vi "LIA Select Decimator.vi"(5 "lock-in.decimator1 0":enum16{"None", "FIR"}(ring), 7 "lock-in.decimator0 0":enum16{"None", "CIC", "FIR", "4HB"}(ring), 8 "error in (no error)":errorcluster, 9 "lock-in.decimation1 0":i32, 10 "lock-in.decimation0 0":i32, 11 "LIA Host Interface in":refnum<class "LIA Host Interface.lvclass">) -> (0 "error out":errorcluster, 3 "LIA Host Interface out":refnum<class "LIA Host Interface.lvclass">)   [LabVIEW 2017]
uses:
  Program Files (x86)/National Instruments/LabVIEW 2017/examples/Lock-In Amplifier/lib/interface/Interface/LIA Host Interface.lvclass
  Program Files (x86)/National Instruments/LabVIEW 2017/examples/Lock-In Amplifier/lib/interface/Interface FPGA/LIA Host Interface FPGA.lvclass
  Program Files (x86)/National Instruments/LabVIEW 2017/examples/Lock-In Amplifier/lib/host/Public/fpga type.ctl
  Program Files (x86)/National Instruments/LabVIEW 2017/examples/Lock-In Amplifier/lib/interface/Interface FPGA/Properties/FpgaSession_GET.vi
  <vilib>/Utility/error.llb/Error Cluster From Error Code.vi
  <vilib>/rvi/errors/niLvFpgaAdjustHostInterfaceError.vi
  <vilib>/rvi/interface/nirviReadWriteControl/nirviReadWriteControl.xnode
  Program Files (x86)/National Instruments/LabVIEW 2017/examples/Lock-In Amplifier/lib/host/Lock-In Amplifier Example Host.lvlib
  NiFpgaLv.dll
  <vilib>/rvi/interface/Simulation/niFpgaSimulationCallBeginRW.vi
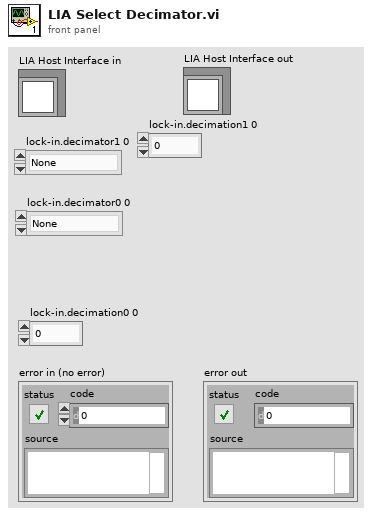
[diagram p1: front panel]
types:
  T1 = typedef "Lock-In Amplifier Example Host.lvlib/fpga type.ctl" = refnum<k20>
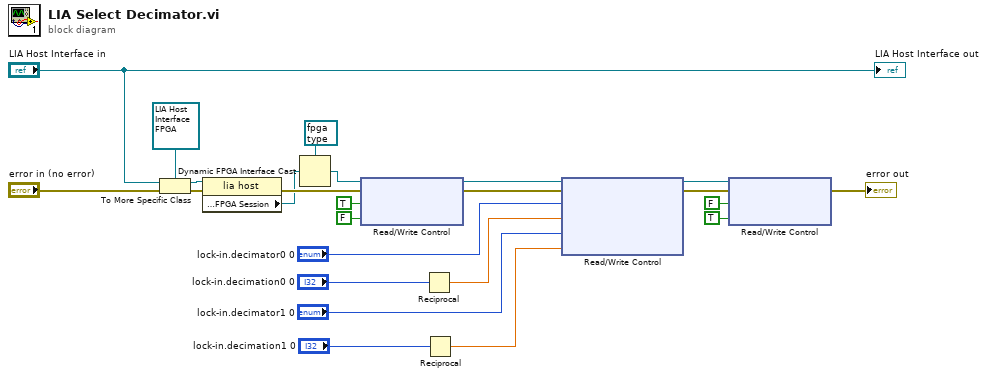
[diagram p0: block diagram]
diagram:
  n1 = To More Specific Class(target class=refnum<class "LIA Host Interface FPGA.lvclass"> refnum ("lia host"), reference="LIA Host Interface in", error in="error in (no error)") -> (specific class reference=w19:refnum<class "LIA Host Interface FPGA.lvclass">, error out=w18:errorcluster)
  n2 = property class="lia host"(reference=w19, error in=w18) -> (error out=w24:errorcluster, "Properties:FPGA Session"=w20:refnum<k20>)  [unwired: 1 out]
  n3 = Dynamic FPGA Interface Cast(Session In=T1 refnum ("fpga type"), Type=w20) -> (Session Out=w12:T1)
  n4 = xnode "Read/Write Control"("FPGA VI Reference In"=w12, "error in"=w24, "lock-in.reset 0"=TRUE, "lock-in.enable 0"=FALSE) -> ("FPGA VI Reference Out"=w11:T1, "error out"=w13:errorcluster)
  n5 = Reciprocal(x="lock-in.decimation0 0") -> (1/x=w23:dbl)
  n6 = Reciprocal(x="lock-in.decimation1 0") -> (1/x=w1:dbl)
  n7 = xnode "Read/Write Control"("FPGA VI Reference In"=w11, "error in"=w13, "lock-in.decimator 0"="lock-in.decimator0 0", "lock-in.fir fs"=w23, "lock-in.decimator 1"="lock-in.decimator1 0", "lock-in.fir2 fs"=w1) -> ("FPGA VI Reference Out"=w7:T1, "error out"=w22:errorcluster)
  n8 = xnode "Read/Write Control"("FPGA VI Reference In"=w7, "error in"=w22, "lock-in.reset 0"=FALSE, "lock-in.enable 0"=TRUE) -> ("error out"=→"error out":errorcluster)  [unwired: 1 out]
  "LIA Host Interface out" <- "LIA Host Interface in"
